vi "Initialize.vi"(8 "Error in":errorcluster caption="Error in (no error)", 9 "section postfix":string) -> (0 "Error out":errorcluster, 3 "INI-Static-Variable-Support.lvlib:CSM-Static-Variable-Manager.lvclass":refnum<class "CSM-Static-Variable-Manager.lvclass">)   [LabVIEW 2017, in "INI-Static-Variable-Support.lvlib" / "CSM-Static-Variable-Manager.lvclass"]
uses:
  CSM-Static-Variable-Manager.lvclass
  CSM-Static-Variable-Manager.lvclass/CSM-Static-Variable-Manager.ctl
  LabVIEW-Config/LabVIEW-Config.lvclass/LabVIEW-Config.ctl
  LabVIEW-Config/Write Modified.vi
  INI-Static-Variable-Support.lvlib
  LabVIEW-Config/LabVIEW-Config.lvclass
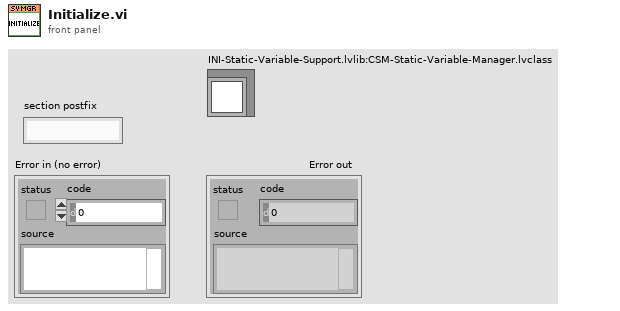
[diagram p1: front panel]
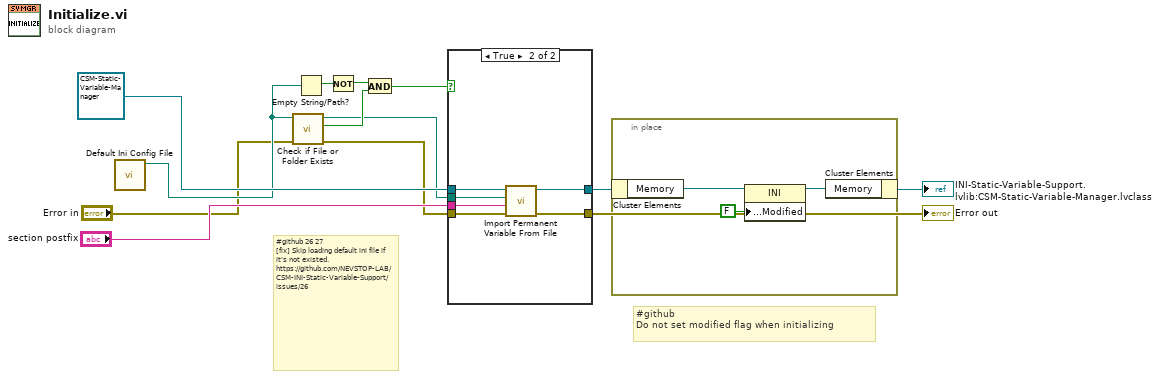
[diagram p0: block diagram]
diagram:
  # "#github\nDo not set modified flag when initializing"
  # "#github 26 27\n[fix] Skip loading default ini file if it's not existed.\nhttps://github.com/NEVSTOP-LAB/CSM-INI-Static-Variable-Support/issues/26"
  n1 = call "Default Ini Config File.vi"() -> ("appended path"=w7:path)  [unwired: 11 in]
  n2 = call <vilib>:"Check if File or Folder Exists.vi"("error in (no error)"="Error in", "path"=w7) -> ("error out"=w5:errorcluster, "file or folder exists?"=w8:bool, "dup path"=w3:path)  [unwired: 7 in]
  n3 = Empty String/Path?(string/path=w7) -> (empty?=w10:bool)
  n4 = Not(x=w10) -> (.not. x?=w9:bool)
  n5 = And(x=w9, y=w8) -> (x .and. y?=w4:bool)
  n6 = case shown="True" w4 {
    tunnel: [w14 w21] -> w13
    tunnel: refnum<class "CSM-Static-Variable-Manager.lvclass"> refnum ("INI-Static-Variable-Support.lvlib:CSM-Static-Variable-Manager.lvclass") -> [w15 w20]
    tunnel: [w15 w19] -> w2
    tunnel: "section postfix" -> [_ w18]
    tunnel: w3 -> [_ w17]
    tunnel: w5 -> [w14 w16]
    frame False {
    }
    frame True {
      n7 = call "Import Permanent Variable From File.vi"("error in (no error)"=w16, "section postfix"=w18, "Path"=w17, "CSM-Static-Variable-Manager in"=w20) -> ("error out"=w21:errorcluster, "CSM-Static-Variable-Manager out"=w19:refnum<class "CSM-Static-Variable-Manager.lvclass">)  [unwired: 6 in]
    }
  }
  "Error out" <- w13
  n8 = in-place {
    n9 = in-place-cluster #1(w2) -> ("Memory"=w24:refnum<class "LabVIEW-Config.lvclass">)
    n10 = property class="INI"(reference=w24, "Properties:Modified"=FALSE ("Modified")) -> (reference out=w23:refnum<class "LabVIEW-Config.lvclass">)  [unwired: 1 in, 1 out]
    n11 = in-place-cluster #1("Memory"=w23) -> (→"INI-Static-Variable-Support.lvlib:CSM-Static-Variable-Manager.lvclass":refnum<class "CSM-Static-Variable-Manager.lvclass">)
  }
